vi "getOpenPort.vi"() -> (0 "port":u16)   [LabVIEW 2010]
doc: "Returns a local port not currently in use."
uses:
  <userlib>/ROSforLV_0.1/ROS/Code/_ROSDefinition.vi
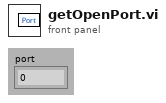
[diagram p1: front panel]
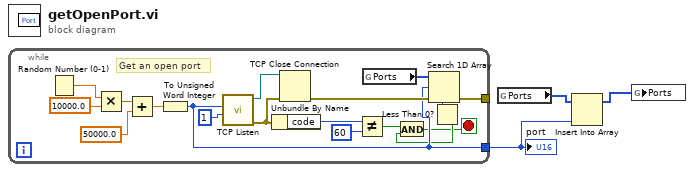
[diagram p0: block diagram]
diagram:
  n1 = while {
    tunnel: [w8] -> w1
    tunnel: [w10] -> _
    stop <- w5 stop-if-true
    # "Get an open port"
    n2 = Random Number (0-1)() -> (number: 0 to 1=w16:dbl)
    n3 = Multiply(x=w16, y=10000.0) -> (x*y=w15:dbl)
    n4 = Add(x=w15, y=50000.0) -> (x+y=w13:dbl)
    n5 = To Unsigned Word Integer(number=w13) -> (unsigned 16bit integer=w8:u16)
    n6 = call <vilib>:"TCP Listen.vi"("timeout ms (wait forever: -1)"=1, "port"=w8) -> ("error out"=w11:errorcluster, "connection ID"=w12:refnum<k5>)  [unwired: 6 in, 2 out]
    n7 = Unbundle By Name(w11) -> ("code"=w19:i32)
    n8 = TCP Close Connection(connection ID=w12, error in (no error)=w11) -> (error out=w10:errorcluster)  [unwired: 1 in, 1 out]
    n9 = Not Equal?(x=w19, y=60) -> (x != y?=w4:bool)
    n10 = global read "_ROSDefinition.vi" "Ports"() -> (w9:u16[])
    n11 = Search 1D Array(1D array=w9, element=w8) -> (index of element=w7:i32)  [unwired: 1 in]
    n12 = Less Than 0?(x=w7) -> (x < 0?=w6:bool)
    n13 = And(x=w4, y=w6) -> (x .and. y?=w5:bool)
  }
  "port" <- w1
  n14 = global read "_ROSDefinition.vi" "Ports"() -> (w3:u16[])
  n15 = Insert Into Array(array=w3, new element=w1) -> (w2:u16[])  [unwired: 1 in]
  n16 = global write "_ROSDefinition.vi" "Ports"(w2) -> ()
